vi "wait_with_error_conections.vi"(8 "error in (no error)":errorcluster, 11 "milliseconds to wait":u32=300) -> (0 "error out":errorcluster)   [LabVIEW 2023]
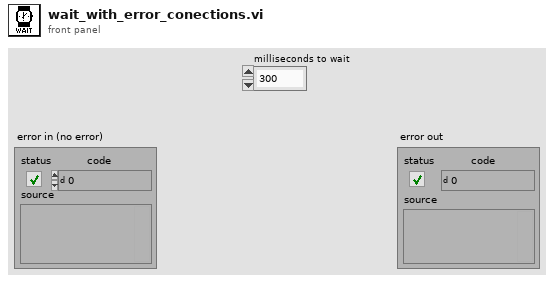
[diagram p1: front panel]
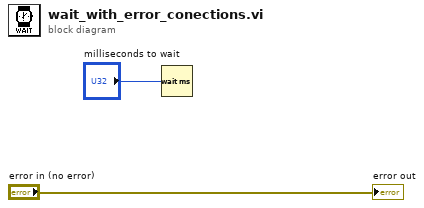
[diagram p0: block diagram]
diagram:
  n1 = Wait (ms)(milliseconds to wait="milliseconds to wait") -> ()  [unwired: 1 out]
  "error out" <- "error in (no error)"
